vi "Read Transfer Group Buffer.vi"(8 "error in (no error)":errorcluster, 10 "Transfer Group":refnum<class "Transfer Group.lvclass">, 11 "UDP Transceiver in":refnum<class "UDP Transceiver.lvclass">) -> (0 "error out":errorcluster, 1 "data":string, 3 "UDP Transceiver out":refnum<class "UDP Transceiver.lvclass">)   [LabVIEW 2017, in "UDP.lvlib" / "UDP Transceiver.lvclass"]
uses:
  UDP Transceiver.lvclass
  Builds/Data Sharing Framework/Current/Core/DSF Core.lvlibp/Classes/Transfer Group/Transfer Group.lvclass
  UDP Transceiver.lvclass/UDP Transceiver.ctl
  Builds/Data Sharing Framework/Current/Core/DSF Core.lvlibp/Classes/Buffer/Read Buffer 1D U8.vi
  Builds/Data Sharing Framework/Current/Core/DSF Core.lvlibp/Classes/Buffer/Buffer.lvclass
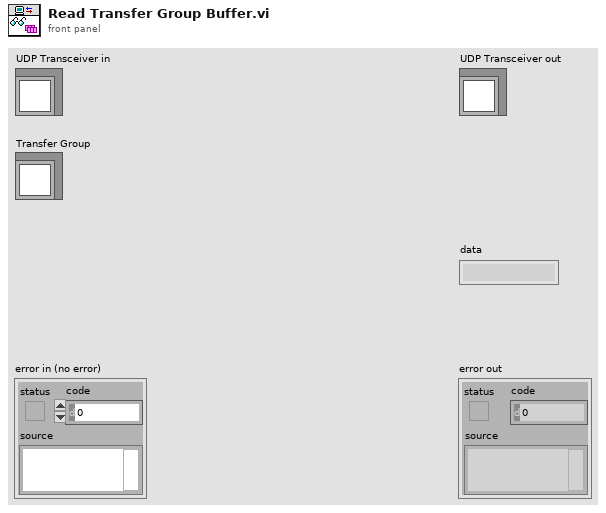
[diagram p1: front panel]
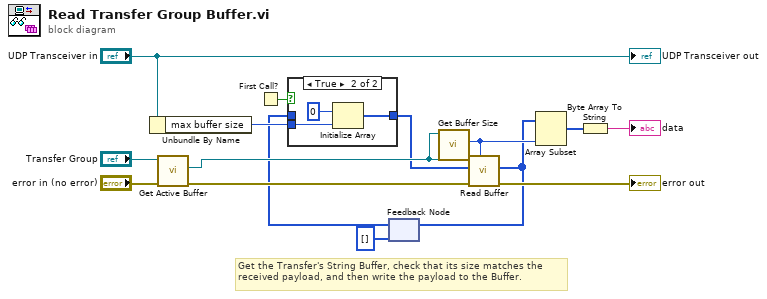
[diagram p0: block diagram]
diagram:
  # "Get the Transfer's String Buffer, check that its size matches the received payload, and then write the payload to the Buffer."
  n1 = Unbundle By Name("UDP Transceiver in") -> ("max buffer size"=w4:u64)
  n2 = call "Get Active Buffer.vi"("error in (no error)"="error in (no error)", "Transfer Group in"="Transfer Group") -> ("error out"=w11:errorcluster, "Buffer"=w3:refnum<class "Buffer.lvclass">)  [unwired: 7 in, 1 out]
  n3 = First Call?() -> (First Call?: T/F=w6:bool)
  n4 = feedback #1(u8[] []) -> (w1:u8[])
  n5 = case shown="True" w6 {
    tunnel: w1 -> [w16 _]
    tunnel: [w16 w19] -> w2
    tunnel: w4 -> [_ w17]
    frame False {
    }
    frame True {
      n6 = Initialize Array(u8 0 ("Numeric"), w17) -> (w19:u8[])
    }
  }
  n7 = call "Get Buffer Size.vi"("Buffer in"=w3) -> ("buffer size"=w10:u64)  [unwired: 9 in, 1 out]
  n8 = call-poly "Read Buffer.vi"("count (-1: rest)"=w10, "error in (no error)"=w11, "dst array in"=w2, "Buffer in"=w3) -> ("error out"=→"error out":errorcluster, "dst array out"=w5:u8[])  [unwired: 4 in, 2 out]
  n9 = feedback-in #1(w5) -> ()
  n10 = Array Subset(array=w5, length=w10) -> (w13:u8[])  [unwired: 1 in]
  n11 = Byte Array To String(unsigned byte array=w13) -> (string=→"data":string)
  "UDP Transceiver out" <- "UDP Transceiver in"
